vi "Test.vi"() -> ()   [LabVIEW 2018, in "TestSlave.lvlib"]
uses:
  TestSlave.lvlib
  Loop Control.xctl
  Test Sensor.xctl
  <vilib>/Platform/TimedLoop/XDataNode/timing_clust.ctl
  <vilib>/Platform/TimedLoop/XDataNode/nitl_modes.ctl
  <vilib>/Platform/TimedLoop/XDataNode/wakeup.ctl
  <vilib>/platform/TimedLoop/XDataNode/XDataNode.xnode
  <vilib>/Platform/TimedLoop/XDataNode/XDNodeRunTimeDep.lvlib
panel:
  out "Waveform Chart":sgl[](graph)
  in  "Second":T1(xcontrol)
  in  "Main":T1(xcontrol)
  in  "Loop Control":T2(xcontrol)
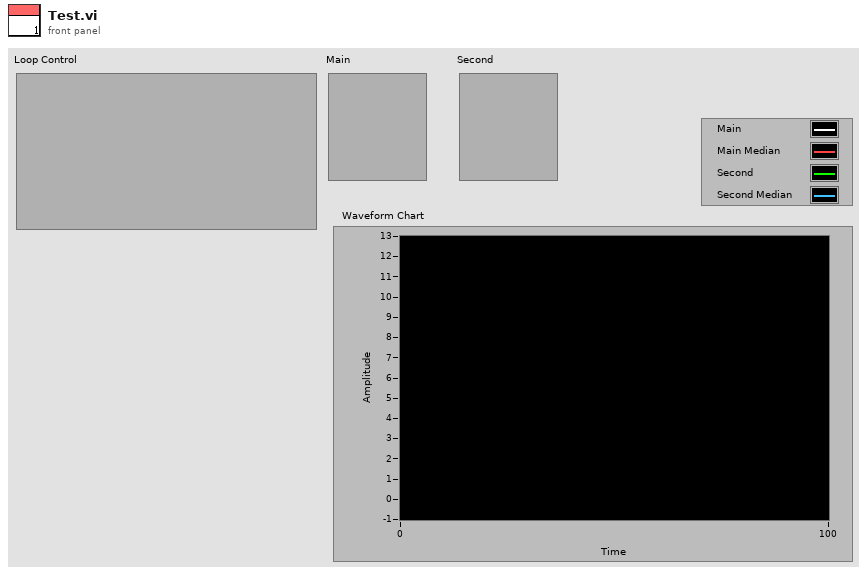
[diagram p1: front panel]
types:
  T1 = cluster{"Status":enum8{"Undefined", "Operational", "Above Range", "Below Range", "Fault"}, "Code":u8}
  T2 = cluster{"dt":i64, "error to show":errorcluster, "Active":bool, "stop":bool}
  T3 = typedef "XDNodeRunTimeDep.lvlib/timing_clust.ctl" = cluster{"Expected End [f-1]":u64, "Actual End [f-1]":u64, "Finished Late? [f-1]":bool, "Expected End [i-1]":u64, "Actual End [i-1]":u64, "Finished Late? [i-1]":bool, "Expected Start [i]":u64, "Actual Start [i]":u64, "Expected Start [f]":u64, "Actual Start [f]":u64, "Source Name":string, "Structure Name":string, "Period":i64, "Deadline":i64, "Offset":i64, "Start":i64, "Priority":i32, "Timeout":i32, "Mode":T4, "Wakeup Reason":T5, "Error":errorcluster, "Source Type":string, "Secondary Source Type":string, "Global End Time":u64, "Global Start Time":u64, "Frame Duration":u64, "Iteration Duration":u64, "Assigned CPU":i32, "I/O Scan Engine Mode":u32}
  T4 = typedef "XDNodeRunTimeDep.lvlib/nitl_modes.ctl" = enum32{"No Change", "Process missed periods, maintain original phase", "Discard missed periods, maintain original phase", "Process missed periods, ignore original phase", "Discard missed periods, ignore original phase"}
  T5 = typedef "XDNodeRunTimeDep.lvlib/wakeup.ctl" = enum32{"Normal", "Aborted", "Asynchronous wakeup", "Timing source error", "Timed loop error", "Timeout"}
  T6 = enum8{"Undefined", "Operational", "Above Range", "Below Range", "Fault"}
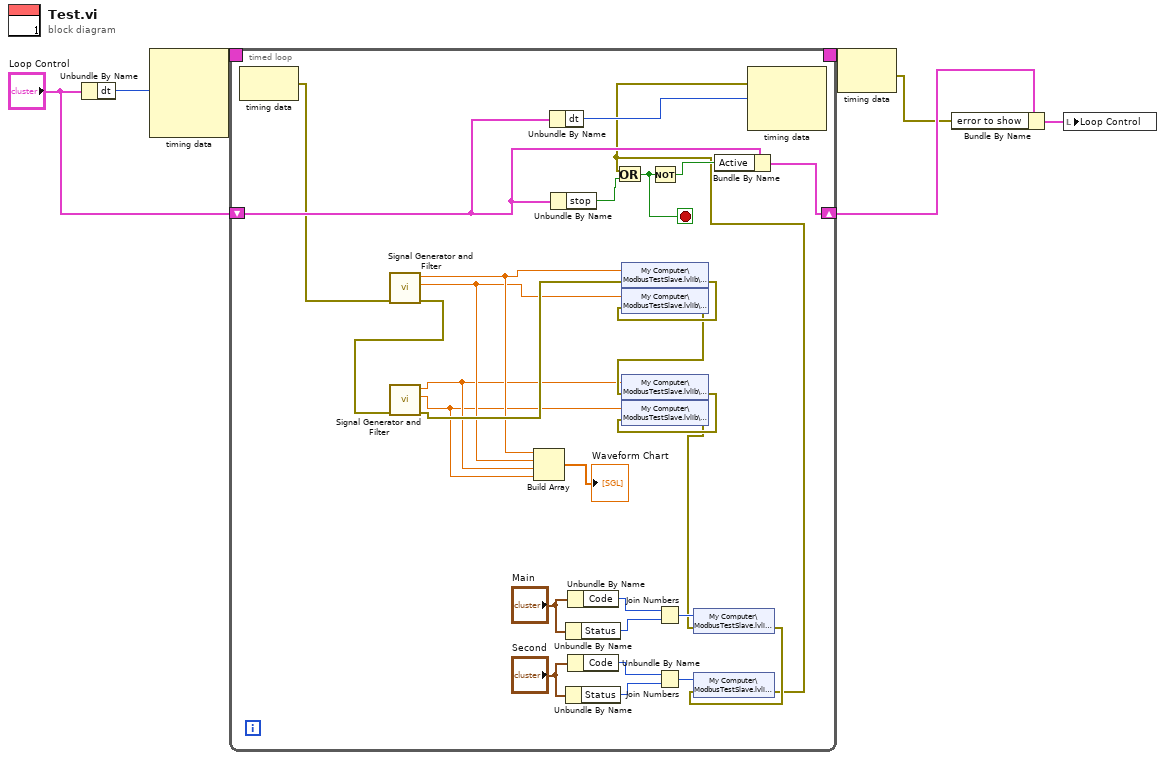
[diagram p0: block diagram]
diagram:
  n1 = Unbundle By Name("Loop Control") -> ("dt"=w5:i64)
  n2 = node-c288(w5) -> (w7:T3)  [unwired: 3 in]
  n3 = timed-loop {
    timing: w7 -> [_]
    timing-out: [_] -> w6
    shift-right: [w31] -> w3
    shift-left: "Loop Control" -> [w34]
    stop <- w32 stop-if-true
    n4 = node-c288() -> (w29:errorcluster)  [unwired: 1 in]
    n5 = call "Signal Generator and Filter.vi"("error in (no error)"=w29) -> ("error out"=w20:errorcluster, "Numeric"=w11:sgl, "Numeric 2"=w12:sgl)  [unwired: 8 in]
    n6 = call "Signal Generator and Filter.vi"("error in (no error)"=w20) -> ("error out"=w19:errorcluster, "Numeric"=w9:sgl, "Numeric 2"=w10:sgl)  [unwired: 8 in]
    n7 = Build Array(w12, w11, w10, w9) -> (→"Waveform Chart":sgl[])
    n8 = Unbundle By Name(w34) -> ("dt"=w30:i64)
    n9 = Unbundle By Name(w34) -> ("stop"=w35:bool)
    n10 = Unbundle By Name("Main") -> ("Status"=w25:T6)
    n11 = Unbundle By Name("Second") -> ("Status"=w21:T6)
    n12 = Unbundle By Name("Main") -> ("Code"=w26:u8)
    n13 = Unbundle By Name("Second") -> ("Code"=w22:u8)
    n14 = shared-variable "My Computer\\ModbusTestSlave.lvlib\\F300006"(w12, error in=w19) -> (error out=w18:errorcluster)
    n15 = shared-variable "My Computer\\ModbusTestSlave.lvlib\\F300006"(w11, error in=w18) -> (error out=w17:errorcluster)
    n16 = shared-variable "My Computer\\ModbusTestSlave.lvlib\\F300011"(w10, error in=w17) -> (error out=w16:errorcluster)
    n17 = shared-variable "My Computer\\ModbusTestSlave.lvlib\\F300013"(w9, error in=w16) -> (error out=w15:errorcluster)
    n18 = Join Numbers(hi=w26, lo=w25) -> ((hi.lo)=w24:u16)
    n19 = Join Numbers(hi=w22, lo=w21) -> ((hi.lo)=w23:u16)
    n20 = shared-variable "My Computer\\ModbusTestSlave.lvlib\\300001"(w24, error in=w15) -> (error out=w14:errorcluster)
    n21 = shared-variable "My Computer\\ModbusTestSlave.lvlib\\300005"(w23, error in=w14) -> (error out=w13:errorcluster)
    n22 = Or(x=w13, y=w35) -> (x .or. y?=w32:bool)
    n23 = Not(x=w32) -> (.not. x?=w33:bool)
    n24 = Bundle By Name(cluster=w34, "Active"=w33) -> (w31:T2)
    n25 = node-c288(w13, w30) -> ()  [unwired: 1 in, 1 out]
  }
  n26 = node-c288(w6) -> (w2:errorcluster)
  n27 = Bundle By Name(cluster=w3, "error to show"=w2) -> (w1:T2)
  n28 = local write "Loop Control"(w1) -> ()
